vi "Color_detection_ROI_tools.vi"() -> ()   [LabVIEW 2025]
uses:
  <vilib>/vision/NI_Vision_Development_Module.lvlib
panel:
  in  "Global Rectangle 2":i32[](array[numeric])
  out "Extracted ROI":T1(plugin-control)
  in  "Enum":enum16{"Color detection", "ROI extraction"}(ring)
  out "Color":u32(colorbox)
  out "B":u8
  out "G":u8
  out "R":u8
  out "Pixel Value (I16)":u32
  in  "X Coordinate":i32
  in  "Y Coordinate":i32
  out "Image":T1(plugin-control)
  in  "File Path":path
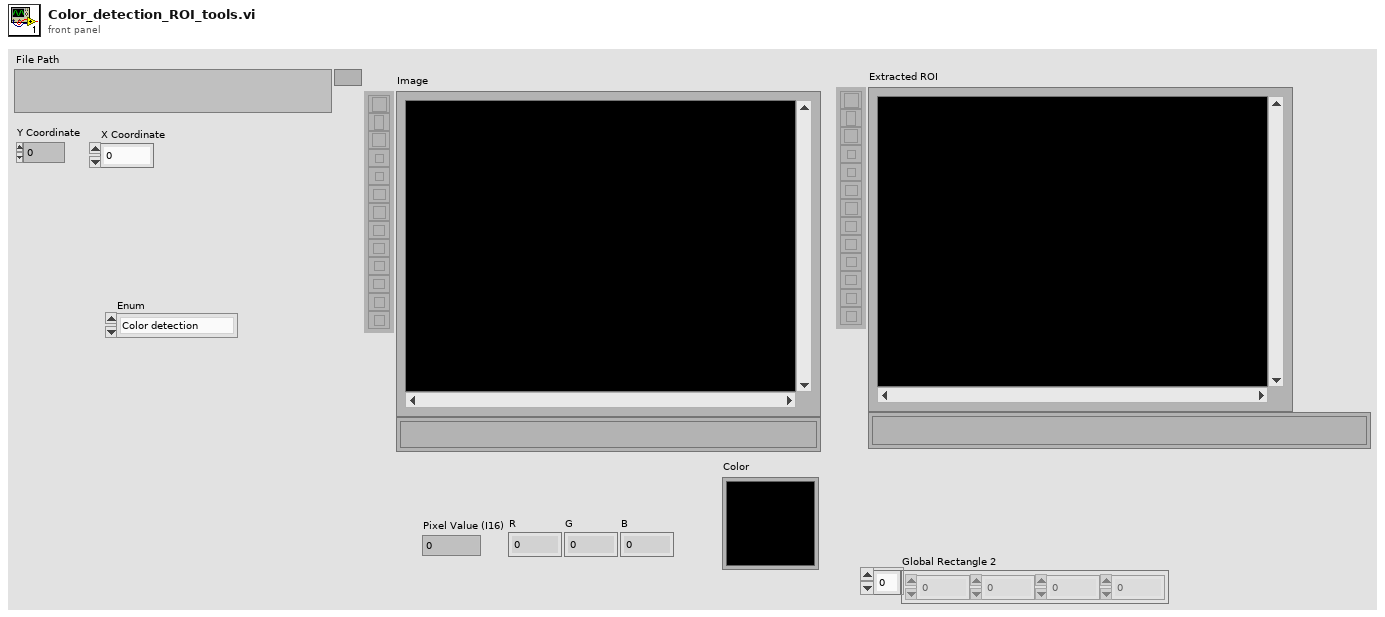
[diagram p1: front panel]
types:
  T1 = typedef "IMAQ Image.ctl" = refnum<image>
  T2 = typedef "Image Type" = u32
  T3 = cluster{"Global Rectangle":i32[], "Contours":cluster{"Contour Type":u32, "ROI Type":u32, "Points":i32[]}[]}
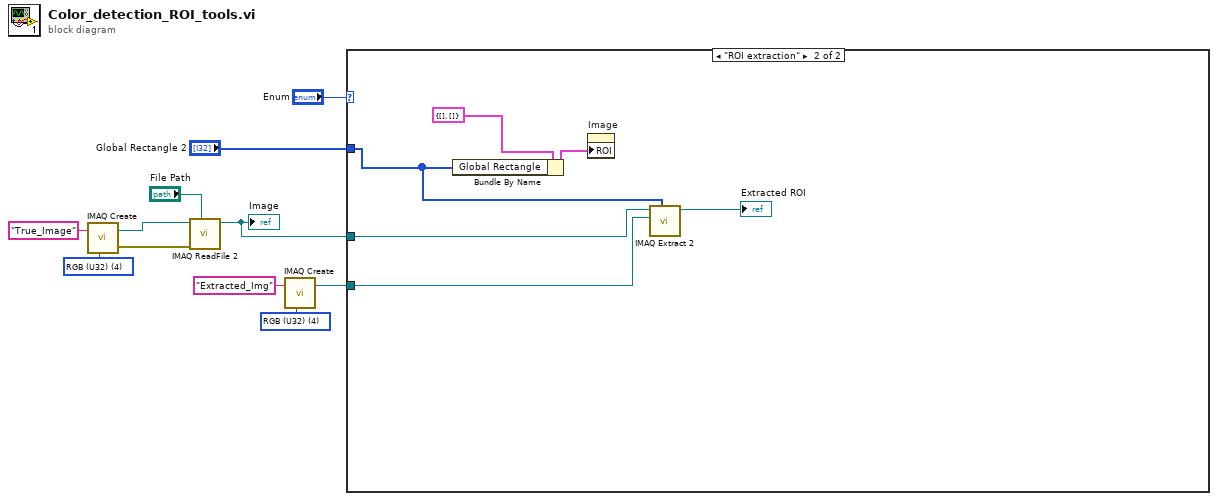
[diagram p0: block diagram]
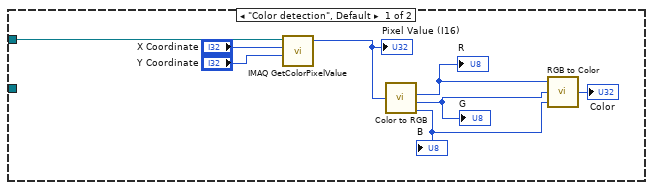
[diagram p2: hidden frame]
diagram:
  w3 = T2 4 items=["Grayscale (U8)", "Grayscale (I16)", "Grayscale (SGL)", "Complex (CSG)", "RGB (U32)", "HSL (U32)", "RGB (U64)", "Grayscale (U16)"] ("Image Type")
  w10 = T2 4 items=["Grayscale (U8)", "Grayscale (I16)", "Grayscale (SGL)", "Complex (CSG)", "RGB (U32)", "HSL (U32)", "RGB (U64)", "Grayscale (U16)"] ("Image Type")
  n1 = call "IMAQ Create"("Image Name"="True_Image", "Image Type"=w10) -> ("New Image"=w8:T1, "error out"=w9:errorcluster)  [unwired: 3 in]
  n2 = call "IMAQ ReadFile 2"("File Path"="File Path", "error in (no error)"=w9, "Image"=w8) -> ("Image Out"=w6:T1)  [unwired: 4 in, 4 out]
  "Image" <- w6
  n3 = call "IMAQ Create"("Image Name"="Extracted_Img", "Image Type"=w3) -> ("New Image"=w2:T1)  [unwired: 3 in, 1 out]
  n4 = case shown="\"ROI extraction\"" "Enum" {
    tunnel: w6 -> [w19 w24]
    tunnel: w2 -> [_ w25]
    tunnel: "Global Rectangle 2" -> [_ w20]
    frame "Color detection", Default {
      n5 = call "IMAQ GetColorPixelValue"("Y Coordinate"="Y Coordinate", "X Coordinate"="X Coordinate", "Image"=w19) -> ("Pixel Value (U32)"=w16:u32)  [unwired: 1 in, 2 out]
      "Pixel Value (I16)" <- w16
      n6 = call <vilib>:"Color to RGB.vi"("Color"=w16) -> ("R"=w15:u8, "G"=w14:u8, "B"=w13:u8)  [unwired: 1 out]
      "R" <- w15
      "G" <- w14
      "B" <- w13
      n7 = call <vilib>:"RGB to Color.vi"("B"=w13, "G"=w14, "R"=w15) -> ("Color"=→"Color":u32)
    }
    frame "ROI extraction" {
      n8 = Bundle By Name(cluster=T3 {"Global Rectangle"=[], "Contours"=[]} ("ROI"), "Global Rectangle"=w20) -> (w21:T3)
      n9 = property on="Image" class="ImageControl"("ROI"=w21) -> ()  [unwired: 2 in, 2 out]
      n10 = call "IMAQ Extract 2"("Optional Rectangle"=w20, "Image Dst"=w25, "Image Src"=w24) -> ("Image Dst Out"=→"Extracted ROI":T1)  [unwired: 7 in, 1 out]
    }
  }
